vi "boolean solo and mute.vi"(11 "Track Controls":T1 {"Track 3"."Volume Settings"."Volume" scale=0.01..10.0; "Track 3"."Volume Settings"."Pan" scale=0.0..1.0; "Track 3"."Effects Settings"."Delay 2" scale=0.0..10.0; "Track 3"."Effects Settings"."Delay" scale=0.0..1.0; "Track 2"."Volume Settings"."Volume" scale=0.01..10.0; "Track 2"."Volume Settings"."Pan" scale=0.0..1.0; "Track 2"."Effects Settings"."Delay 2" scale=0.0..10.0; "Track 2"."Effects Settings"."Delay" scale=0.0..1.0; "Track 1"."Volume Settings"."Volume" scale=0.01..10.0; "Track 1"."Volume Settings"."Pan" scale=0.0..1.0; "Track 1"."Effects Settings"."Delay 2" scale=0.0..10.0; "Track 1"."Effects Settings"."Delay" scale=0.0..1.0; "Track 0"."Volume Settings"."Volume" scale=0.01..10.0; "Track 0"."Volume Settings"."Pan" scale=0.0..1.0; "Track 0"."Effects Settings"."Delay 2" scale=0.0..10.0; "Track 0"."Effects Settings"."Delay" scale=0.0..1.0}) -> (0 "Track 3":bool, 1 "Track 2":bool, 2 "Track 1":bool, 3 "Track 0":bool)   [LabVIEW 2014]
uses:
  Controls/Track Controls.ctl
  Controls/Track Settings.ctl
  Controls/Track Effects Settings.ctl
  Controls/Track Volume Settings.ctl
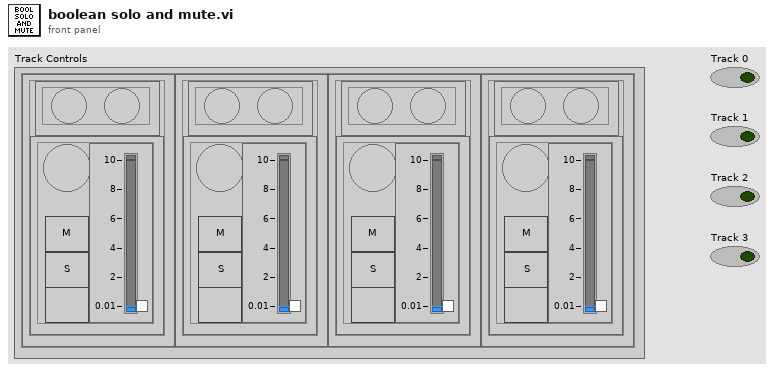
[diagram p1: front panel]
types:
  T1 = typedef "Track Controls.ctl" = cluster{"Track 0":T2, "Track 1":T2, "Track 2":T2, "Track 3":T2}
  T2 = typedef "Track Settings.ctl" = cluster{"Effects Settings":T3, "Volume Settings":T4}
  T3 = typedef "Track Effects Settings.ctl" = cluster{"Delay":dbl, "Delay 2":dbl}
  T4 = typedef "Track Volume Settings.ctl" = cluster{"Mute":bool, "Solo":bool, "Record":bool, "Pan":dbl, "Volume":dbl}
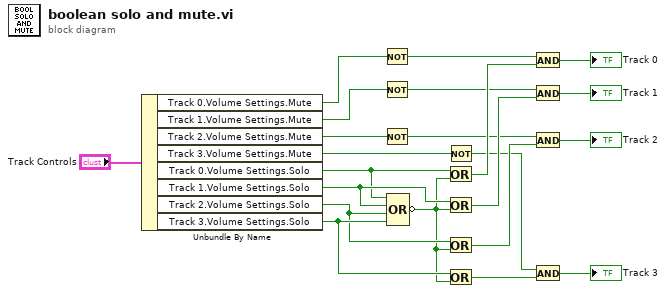
[diagram p0: block diagram]
diagram:
  n1 = Unbundle By Name("Track Controls") -> ("Track 0.Volume Settings.Mute"=w5:bool, "Track 1.Volume Settings.Mute"=w7:bool, "Track 2.Volume Settings.Mute"=w8:bool, "Track 3.Volume Settings.Mute"=w9:bool, "Track 0.Volume Settings.Solo"=w15:bool, "Track 1.Volume Settings.Solo"=w16:bool, "Track 2.Volume Settings.Solo"=w17:bool, "Track 3.Volume Settings.Solo"=w18:bool)
  n2 = Not(x=w5) -> (.not. x?=w6:bool)
  n3 = Not(x=w7) -> (.not. x?=w10:bool)
  n4 = Not(x=w8) -> (.not. x?=w11:bool)
  n5 = Compound Arithmetic op=OR(w15, w16, w17, w18) -> (invert w14:bool)
  n6 = Not(x=w9) -> (.not. x?=w12:bool)
  n7 = Or(x=w15, y=w14) -> (x .or. y?=w19:bool)
  n8 = Or(x=w16, y=w14) -> (x .or. y?=w20:bool)
  n9 = Or(x=w17, y=w14) -> (x .or. y?=w21:bool)
  n10 = Or(x=w18, y=w14) -> (x .or. y?=w22:bool)
  n11 = And(x=w6, y=w19) -> (x .and. y?=→"Track 0":bool)
  n12 = And(x=w10, y=w20) -> (x .and. y?=→"Track 1":bool)
  n13 = And(x=w11, y=w21) -> (x .and. y?=→"Track 2":bool)
  n14 = And(x=w12, y=w22) -> (x .and. y?=→"Track 3":bool)
